vi "Save Data_Corrected.vi"(0 "Experiment Indicator":string, 1 "Username":string, 5 "Pixel":dbl, 7 "Scan direction":i32, 9 "Data Array":dbl[][](array[numeric]), 11 "Cell details cluster":T1={"Measure?"=TRUE, "Area (cm^2)"=0.0, "Cell Label"="", "Cell Description"="", "Cell Position"=0, "Time in rig (s)"=0.0, "Time to next scan (s)"=0.0, "Scan number"=0.0, "When did you stick it in?"=0.0, "Time between scans (s)"=0.0, "Time of the last scan (s)"=0.0, "Scan settings in queue"=0, "Sample Holder"=0.0} {"Scan settings in queue" items=["Regular", "Inverted"]; "Time of the last scan (s)" format="%<%H:%M:%S>t"; "When did you stick it in?" format="%<%H:%M:%S>t"; "Time to next scan (s)" format="%<%H:%M:%S>t"; "Time in rig (s)" format="%<%H:%M:%S>t"}, 12 "Show me Scan \nSettings JV set":T2={"Light Intensity (Suns)"=1.0, "Stabilization Time (s)"=5.0, "Maximum Voltage (V)"=0.0, "Minimum Voltage (V)"=-1.0, "Range Options"=0, "Scan Direction\nDU (T), UD (F)"=TRUE, "Step Size (V)"=0.01, "Source Delay (s)"=0.15} {"Range Options" items=["Auto Range", "Semi-Auto Range", "100 uA", "1 mA", "10 mA", "100 mA", "1A"]}, 13 "Time zero":timestamp) -> (4 "Master Log":string[][](table), 6 "File path for master log":path, 10 "File path for device log":path, 14 "File path for JV data":path, 15 "File path for JV image":path)   [LabVIEW 2011]
uses:
  <vilib>/Utility/file.llb/Write To Spreadsheet File (string).vi
  <vilib>/Utility/file.llb/Read From Spreadsheet File (string).vi
  <vilib>/Analysis/NI_AALPro.lvlib
panel:
  out "PCE":dbl
  out "FF":dbl
  out "Voc":dbl
  out "Jsc":dbl
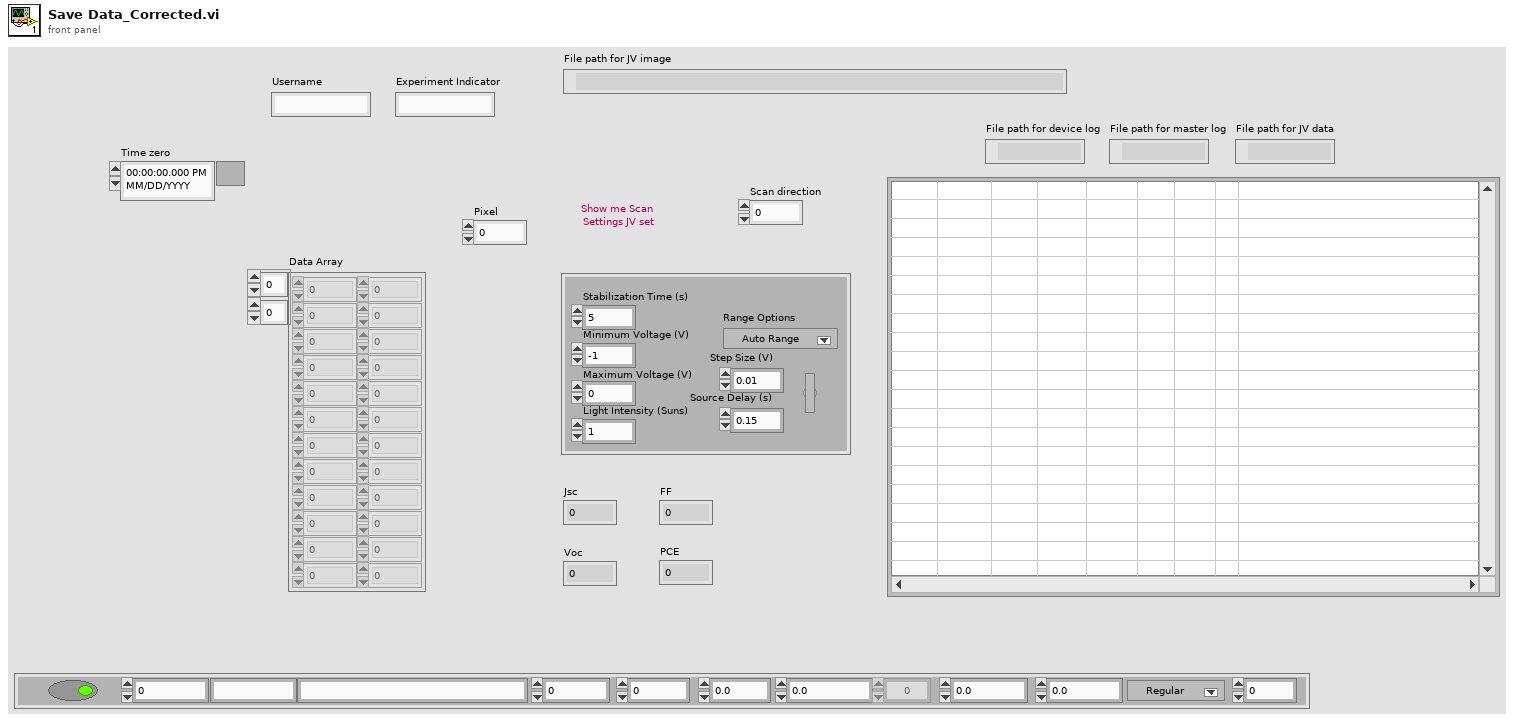
[diagram p1: front panel]
types:
  T1 = cluster{"Measure?":bool, "Area (cm^2)":dbl, "Cell Label":string, "Cell Description":string, "Cell Position":i32, "Time in rig (s)":dbl, "Time to next scan (s)":dbl, "Scan number":dbl, "When did you stick it in?":dbl, "Time between scans (s)":dbl, "Time of the last scan (s)":dbl, "Scan settings in queue":u16, "Sample Holder":dbl}
  T2 = cluster{"Light Intensity (Suns)":dbl, "Stabilization Time (s)":dbl, "Maximum Voltage (V)":dbl, "Minimum Voltage (V)":dbl, "Range Options":u16, "Scan Direction\nDU (T), UD (F)":bool, "Step Size (V)":dbl, "Source Delay (s)":dbl}
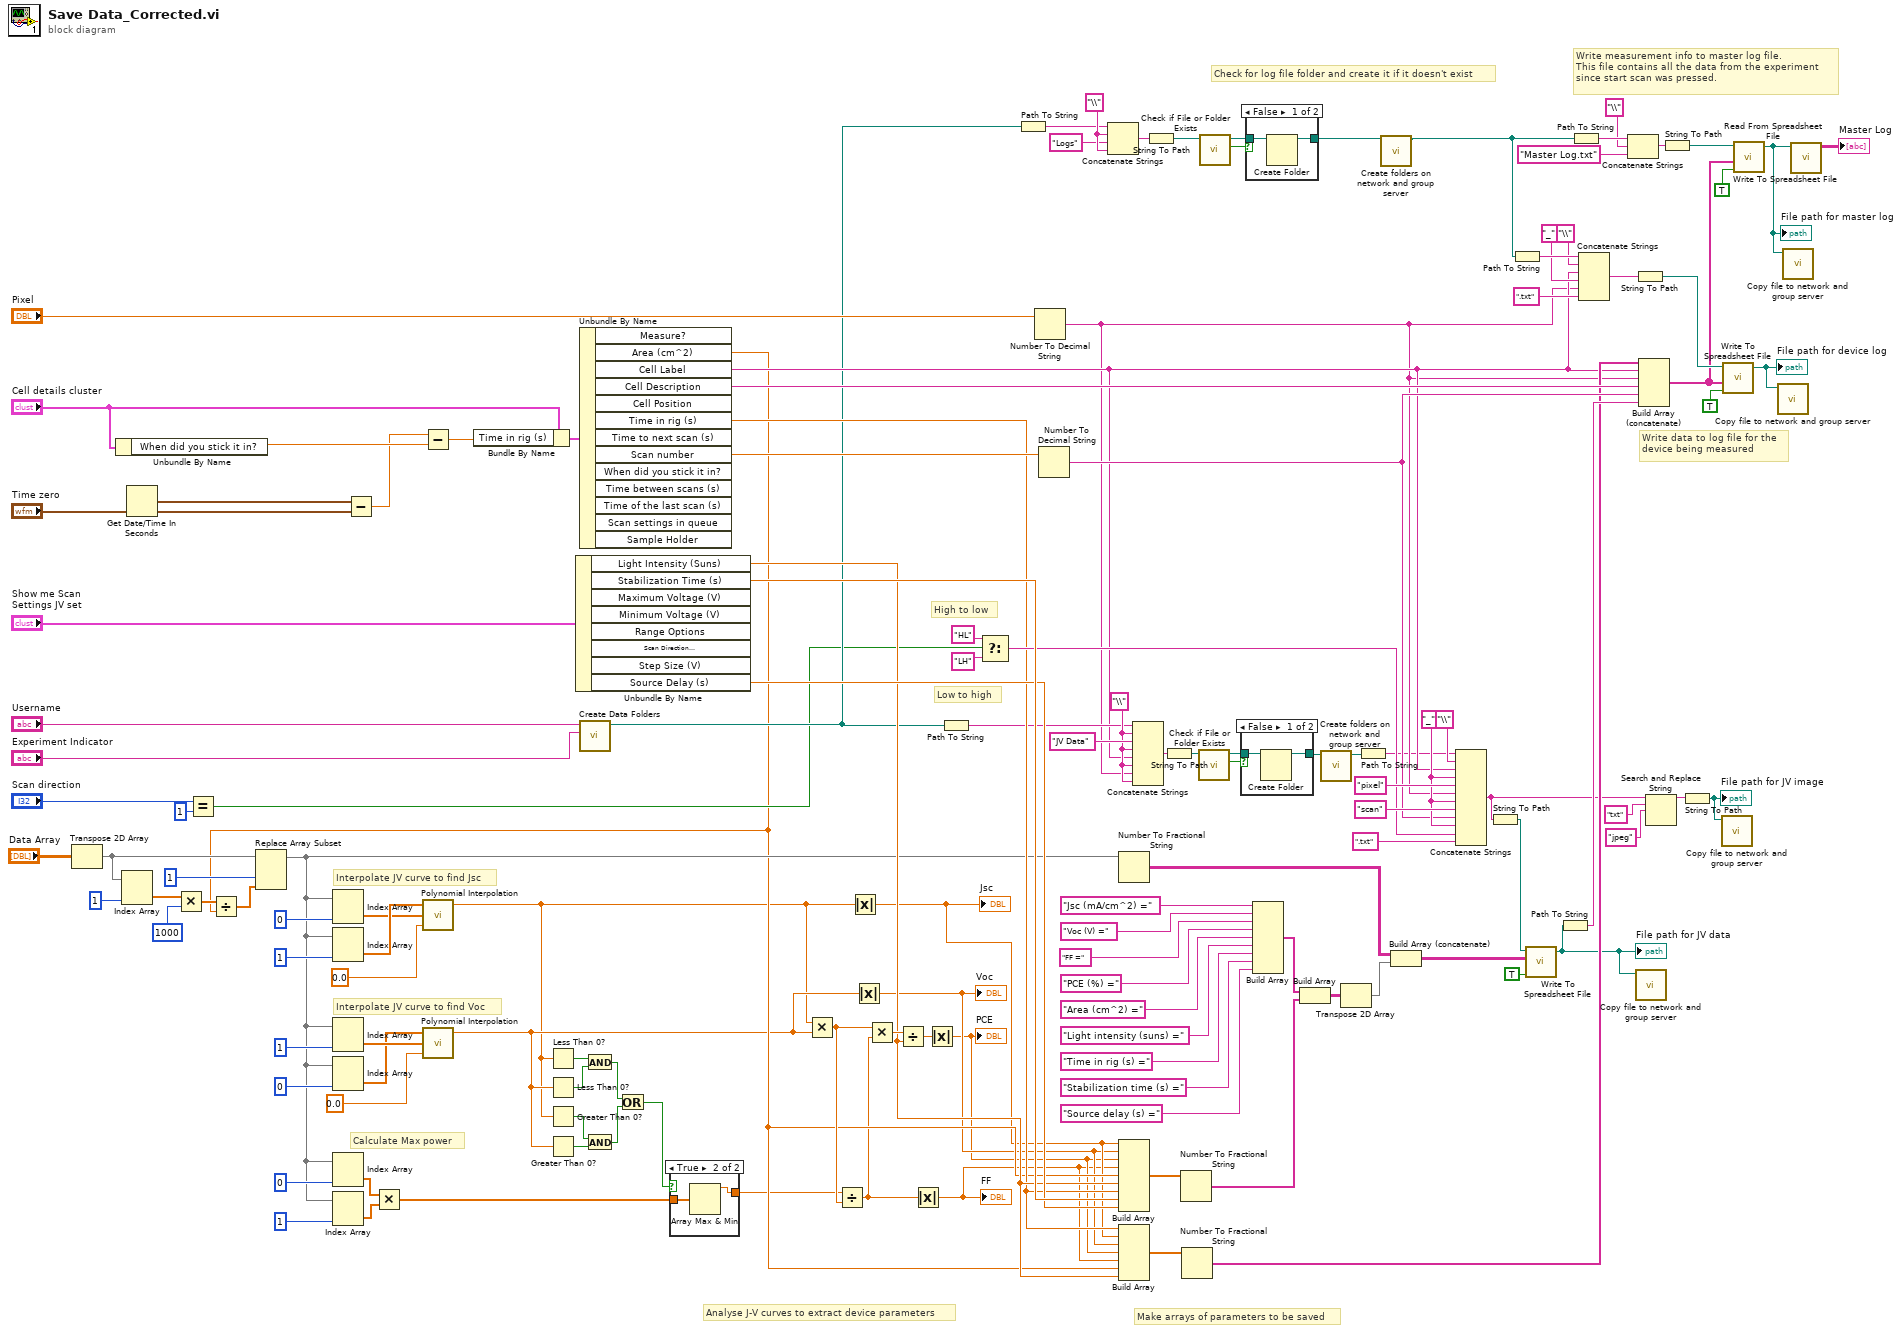
[diagram p0: block diagram]
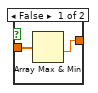
[diagram p2: hidden frame]
diagram:
  w58 = "\\"
  w84 = "\\"
  w97 = "_"
  # "Make arrays of parameters to be saved"
  # "Calculate Max power"
  # "Interpolate JV curve to find Voc"
  # "Interpolate JV curve to find Jsc"
  # "Analyse J-V curves to extract device parameters"
  # "Write data to log file for the\ndevice being measured"
  # "Write measurement info to master log file.\nThis file contains all the data from the experiment\nsince start scan was pressed."
  # "Check for log file folder and create it if it doesn't exist"
  # "Low to high"
  # "High to low"
  n1 = Transpose 2D Array(2D array="Data Array") -> (transposed array=w19:dbl[][])
  n2 = Unbundle By Name("Cell details cluster") -> ("When did you stick it in?"=w42:dbl)
  n3 = Index Array(array=w19, index (col)=1) -> (element=w23:dbl[])  [unwired: 1 in]
  n4 = Get Date/Time In Seconds() -> (seconds since 1Jan1904=w43:timestamp)
  n5 = Multiply(x=w23, y=1000) -> (x*y=w21:dbl[])
  n6 = Equal?(x="Scan direction", y=1) -> (x = y?=w32:bool)
  n7 = Subtract(x=w43, y="Time zero") -> (x-y=w41:dbl)
  n8 = Subtract(x=w41, y=w42) -> (x-y=w39:dbl)
  n9 = Bundle By Name(cluster="Cell details cluster", "Time in rig (s)"=w39) -> (w44:T1)
  n10 = Unbundle By Name("Show me Scan \nSettings JV set") -> ("Light Intensity (Suns)"=w92:dbl, "Stabilization Time (s)"=w107:dbl, "Source Delay (s)"=w106:dbl)  [unwired: 5 out]
  n11 = Unbundle By Name(w44) -> ("Area (cm^2)"=w17:dbl, "Cell Label"=w56:string, "Cell Description"=w90:string, "Time in rig (s)"=w91:dbl, "Scan number"=w102:dbl)  [unwired: 8 out]
  n12 = Divide(x=w21, y=w17) -> (x/y=w20:dbl[])
  n13 = Replace Array Subset(array=w19, new element=w20, index (col)=1) -> (w18:dbl[][])  [unwired: 1 in]
  n14 = Index Array(array=w18, index (col)=0) -> (element=w125:dbl[])  [unwired: 1 in]
  n15 = Index Array(array=w18, index (col)=1) -> (element=w126:dbl[])  [unwired: 1 in]
  n16 = Index Array(array=w18, index (col)=1) -> (element=w124:dbl[])  [unwired: 1 in]
  n17 = Index Array(array=w18, index (col)=0) -> (element=w122:dbl[])  [unwired: 1 in]
  n18 = Index Array(array=w18, index (col)=0) -> (element=w131:dbl[])  [unwired: 1 in]
  n19 = Index Array(array=w18, index (col)=1) -> (element=w130:dbl[])  [unwired: 1 in]
  n20 = Multiply(x=w131, y=w130) -> (x*y=w123:dbl[])
  n21 = call <vilib>:"Polynomial Interpolation.vi"("x value"=0.0, "X"=w125, "Y"=w126) -> ("interpolation value"=w2:dbl)  [unwired: 2 out]
  n22 = call <vilib>:"Polynomial Interpolation.vi"("x value"=0.0, "X"=w124, "Y"=w122) -> ("interpolation value"=w3:dbl)  [unwired: 2 out]
  n23 = Less Than 0?(x=w2) -> (x < 0?=w7:bool)
  n24 = Less Than 0?(x=w3) -> (x < 0?=w4:bool)
  n25 = Greater Than 0?(x=w2) -> (x > 0?=w5:bool)
  n26 = Greater Than 0?(x=w3) -> (x > 0?=w6:bool)
  n27 = call "Create Data Folders.vi"("Experiment Indicator"="Experiment Indicator", "username"="Username") -> ("Data Output Folder"=w50:path)  [unwired: 9 in]
  n28 = And(x=w7, y=w4) -> (x .and. y?=w9:bool)
  n29 = And(x=w5, y=w6) -> (x .and. y?=w8:bool)
  n30 = Or(x=w9, y=w8) -> (x .or. y?=w1:bool)
  n31 = case shown="True" w1 {
    tunnel: w123 -> [w140 w142]
    tunnel: [w139 w141] -> w10
    frame False {
      n32 = Array Max & Min(array=w140) -> (min value=w139:dbl)  [unwired: 3 out]
    }
    frame True {
      n33 = Array Max & Min(array=w142) -> (max value=w141:dbl)  [unwired: 3 out]
    }
  }
  n34 = Multiply(x=w2, y=w3) -> (x*y=w121:dbl)
  n35 = Divide(x=w10, y=w121) -> (x/y=w11:dbl)
  n36 = Absolute Value(x=w2) -> (abs(x)=w16:dbl)
  "Jsc" <- w16
  n37 = Absolute Value(x=w3) -> (abs(x)=w15:dbl)
  "Voc" <- w15
  n38 = Multiply(x=w121, y=w11) -> (x*y=w129:dbl)
  n39 = Divide(x=w129, y=w92) -> (x/y=w14:dbl)
  n40 = Absolute Value(x=w11) -> (abs(x)=w12:dbl)
  "FF" <- w12
  n41 = Absolute Value(x=w14) -> (abs(x)=w13:dbl)
  "PCE" <- w13
  n42 = Path To String(path=w50) -> (string=w57:string)
  n43 = Select(t="HL", s=w32, f="LH") -> (s? t:f=w96:string)
  n44 = Path To String(path=w50) -> (string=w81:string)
  n45 = Number To Decimal String(number="Pixel") -> (decimal integer string=w55:string)  [unwired: 1 in]
  n46 = Number To Decimal String(number=w102) -> (decimal integer string=w89:string)  [unwired: 1 in]
  n47 = Concatenate Strings(w81, w84, "Logs", w84) -> (w82:string)
  n48 = Number To Fractional String(number=w18) -> (F-format string=w35:string[][])  [unwired: 3 in]
  n49 = Build Array(w16, w15, w13, w12, w17, w92, w91, w107, w106) -> (w116:dbl[])
  n50 = Build Array(w91, w16, w15, w13, w12, w17, w92) -> (w87:dbl[])
  n51 = Concatenate Strings(w57, w58, "JV Data", w58, w56, w58, w55, w58) -> (w62:string)
  n52 = String To Path(string=w82) -> (path=w80:path)
  n53 = String To Path(string=w62) -> (path=w61:path)
  n54 = Number To Fractional String(number=w116) -> (F-format string=w114:string[])  [unwired: 3 in]
  n55 = Number To Fractional String(number=w87) -> (F-format string=w86:string[])  [unwired: 3 in]
  n56 = call <vilib>:"Check if File or Folder Exists.vi"("path"=w61) -> ("file or folder exists?"=w60:bool, "dup path"=w59:path)  [unwired: 8 in, 1 out]
  n57 = call <vilib>:"Check if File or Folder Exists.vi"("path"=w80) -> ("file or folder exists?"=w79:bool, "dup path"=w78:path)  [unwired: 8 in, 1 out]
  n58 = case shown="False" w60 {
    tunnel: w59 -> [w144 w145]
    tunnel: [w143 w145] -> w28
    frame False {
      n59 = Create Folder(path (use dialog)=w144) -> (created path=w143:path)  [unwired: 2 in, 2 out]
    }
    frame True {
    }
  }
  n60 = case shown="False" w79 {
    tunnel: w78 -> [w147 w148]
    tunnel: [w146 w148] -> w30
    frame False {
      n61 = Create Folder(path (use dialog)=w147) -> (created path=w146:path)  [unwired: 2 in, 2 out]
    }
    frame True {
    }
  }
  n62 = Build Array("Jsc (mA/cm^2) =", "Voc (V) =", "FF =", "PCE (%) =", "Area (cm^2) =", "Light intensity (suns) =", "Time in rig (s) =", "Stabilization time (s) =", "Source delay (s) =") -> (w115:string[])
  n63 = Build Array(w115, w114) -> (w105:string[][])
  n64 = call "Create folders on network and group server.vi"("File path in"=w28) -> ("File path out"=w27:path)  [unwired: 10 in]
  n65 = Transpose 2D Array(2D array=w105) -> (transposed array=w104:string[][])
  n66 = Path To String(path=w27) -> (string=w54:string)
  n67 = call "Create folders on network and group server.vi"("File path in"=w30) -> ("File path out"=w29:path)  [unwired: 10 in]
  n68 = Build Array (concatenate)(w35, w104) -> (w113:string[][])
  n69 = Concatenate Strings(w54, "\\", w56, w97, "pixel", w55, w97, "scan", w89, w97, w96, ".txt") -> (w53:string)
  n70 = String To Path(string=w53) -> (path=w94:path)
  n71 = Path To String(path=w29) -> (string=w77:string)
  n72 = call-poly <vilib>:"Write To Spreadsheet File.vi"("append to file? (new file:F)"=TRUE, "2D data"=w113, "file path (dialog if empty)"=w94) -> ("new file path (Not A Path if cancelled)"=w26:path)  [unwired: 5 in]
  "File path for JV data" <- w26
  n73 = Path To String(path=w26) -> (string=w88:string)
  n74 = Path To String(path=w29) -> (string=w73:string)
  n75 = Concatenate Strings(w77, "\\", w56, "_", w55, ".txt") -> (w75:string)
  n76 = Concatenate Strings(w73, "\\", "Master Log.txt") -> (w70:string)
  n77 = String To Path(string=w75) -> (path=w74:path)
  n78 = call "Copy file to network and group server.vi"("File path in"=w26) -> ()  [unwired: 11 in]
  n79 = Build Array (concatenate)(w86, w56, w55, w90, w89, w88) -> (w68:string[])
  n80 = Search and Replace String(input string=w53, search string="txt", replace string="jpeg") -> (result string=w52:string)  [unwired: 5 in, 3 out]
  n81 = String To Path(string=w70) -> (path=w69:path)
  n82 = String To Path(string=w52) -> (path=w47:path)
  "File path for JV image" <- w47
  n83 = call "Copy file to network and group server.vi"("File path in"=w47) -> ()  [unwired: 11 in]
  n84 = call-poly <vilib>:"Write To Spreadsheet File.vi"("append to file? (new file:F)"=TRUE, "1D data"=w68, "file path (dialog if empty)"=w74) -> ("new file path (Not A Path if cancelled)"=w46:path)  [unwired: 5 in]
  "File path for device log" <- w46
  n85 = call-poly <vilib>:"Write To Spreadsheet File.vi"("append to file? (new file:F)"=TRUE, "1D data"=w68, "file path (dialog if empty)"=w69) -> ("new file path (Not A Path if cancelled)"=w45:path)  [unwired: 5 in]
  "File path for master log" <- w45
  n86 = call "Copy file to network and group server.vi"("File path in"=w46) -> ()  [unwired: 11 in]
  n87 = call "Copy file to network and group server.vi"("File path in"=w45) -> ()  [unwired: 11 in]
  n88 = call-poly <vilib>:"Read From Spreadsheet File.vi"("file path (dialog if empty)"=w45) -> ("all rows"=→"Master Log":string[][])  [unwired: 6 in, 4 out]
